vi "Remove Duplicate Entries in Sorted 1D Array LV2012 NI Verified.vi"(11 "Input":string[](array[string])=["A", "A", "A"]) -> (3 "Output":string[](array[string]))   [LabVIEW 2018]
doc: "Use this VI to remove duplicate, adjacent elements from an array. To use this VI, enter values in the \"In\" array and run."
panel:
  # "Overview: This VI removes duplicate adjacent entries in a 1D array. If entries are not adjacent ,they will not be removed\nRequirements: LabVIEW 2012 (or compatible)\nInstructions:\n1. Manually Initialize the Input Array \n2. Run the VI\n3. To display Help for this VI, Select Help»Show Context Help and move the cursor over the VI icon to display help for this VI"
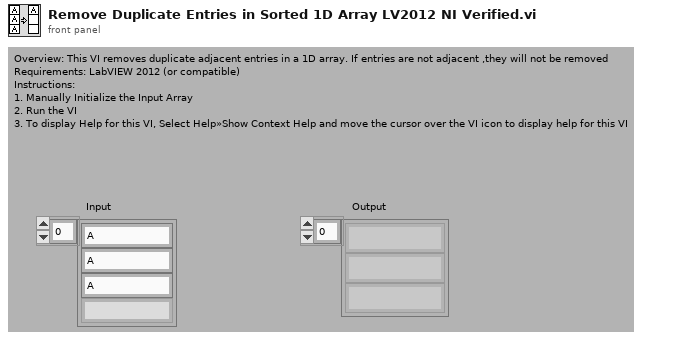
[diagram p1: front panel]
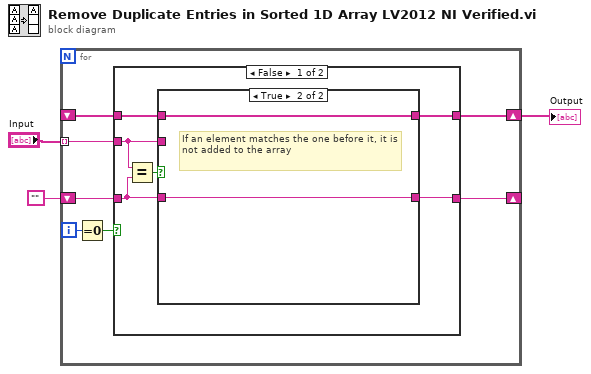
[diagram p0: block diagram]
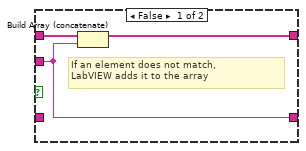
[diagram p2: hidden frame]
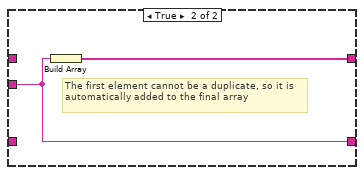
[diagram p3: hidden frame]
diagram:
  n1 = for {
    tunnel: "Input" -> [w8] mode=indexing
    shift-right: [w6] -> _
    shift-left: "" -> [w5]
    shift-right: [w7] -> w2
    shift-left: _ -> [w4]
    i -> [w10]
    n2 = Equal To 0?(x=w10) -> (x = 0?=w9:bool)
    n3 = case shown="False" w9 {
      tunnel: w8 -> [w13 w22]
      tunnel: [w14 w23] -> w7
      tunnel: [w16 w22] -> w6
      tunnel: w5 -> [w12 _]
      tunnel: w4 -> [w15 _]
      frame False {
        n4 = Equal?(x=w13, y=w12) -> (x = y?=w11:bool)
        n5 = case shown="True" w11 {
          tunnel: w12 -> [_ w21]
          tunnel: [w17 w21] -> w16
          tunnel: [w18 w20] -> w14
          tunnel: w15 -> [w19 w20]
          tunnel: w13 -> [w17 _]
          frame False {
            # "If an element does not match,\nLabVIEW adds it to the array"
            n6 = Build Array (concatenate)(w19, w17) -> (w18:string[])
          }
          frame True {
            # "If an element matches the one before it, it is not added to the array"
          }
        }
      }
      frame True {
        # "The first element cannot be a duplicate, so it is automatically added to the final array"
        n7 = Build Array(w22) -> (w23:string[])
      }
    }
  }
  "Output" <- w2
